vi "Path to lvcsm String.vi"(11 "Path":path) -> (3 "Common Path":string)   [LabVIEW 2017, in "lvcsm File Support.lvlib"]
uses:
  lvcsm File Support.lvlib
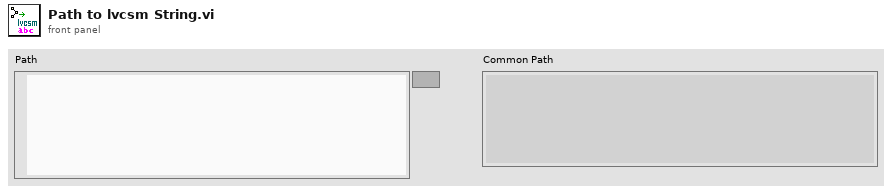
[diagram p1: front panel]
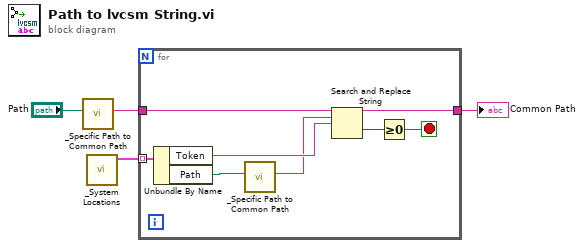
[diagram p0: block diagram]
diagram:
  n1 = call "_Specific Path to Common Path.vi"("Specific Path"="Path") -> ("Common Path"=w1:string)  [unwired: 10 in]
  n2 = call "_System Locations.vi"() -> ("SystemLocations"=w3:cluster{"Token":string, "Path":path}[])  [unwired: 11 in]
  n3 = for {
    tunnel: w1 -> [w12]
    tunnel: [w11] -> w4
    tunnel: w3 -> [w8] mode=indexing
    stop <- w9 stop-if-true
    n4 = Unbundle By Name(w8) -> ("Token"=w7:string, "Path"=w6:path)
    n5 = call "_Specific Path to Common Path.vi"("Specific Path"=w6) -> ("Common Path"=w5:string)  [unwired: 10 in]
    n6 = Search and Replace String(input string=w12, search string=w5, replace string=w7) -> (result string=w11:string, offset past replacement=w10:i32)  [unwired: 5 in, 2 out]
    n7 = Greater Or Equal To 0?(x=w10) -> (x >= 0?=w9:bool)
  }
  "Common Path" <- w4
